vi "motion_control.vi"(2 "position":dbl, 3 "acceleration":dbl, 4 "maxVelocity":dbl, 5 ".NET Refnum in":refnum<k24>) -> (1 ".NET Refnum out":refnum<k24>)   [LabVIEW 2021]
uses:
  C:/Users/User/Documents/Published_files/thorlabs_files/ThorLabs.MotionControl.Benchtop.DCServoCLI.dll
  thorlabs_files/ThorLabs.MotionControl.Benchtop.DCServoCLI.dll
  <vilib>/ptbypt/NI_PtbyPt.lvlib
panel:
  out "end":bool=TRUE
  out "x < y?":bool
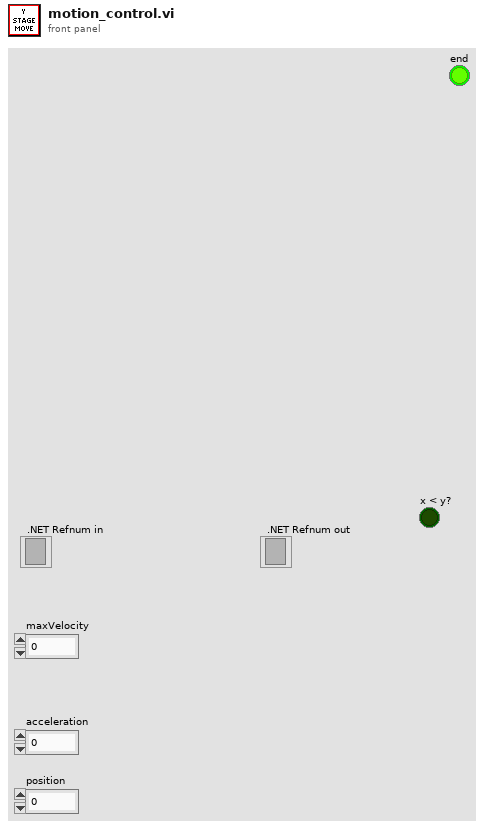
[diagram p1: front panel]
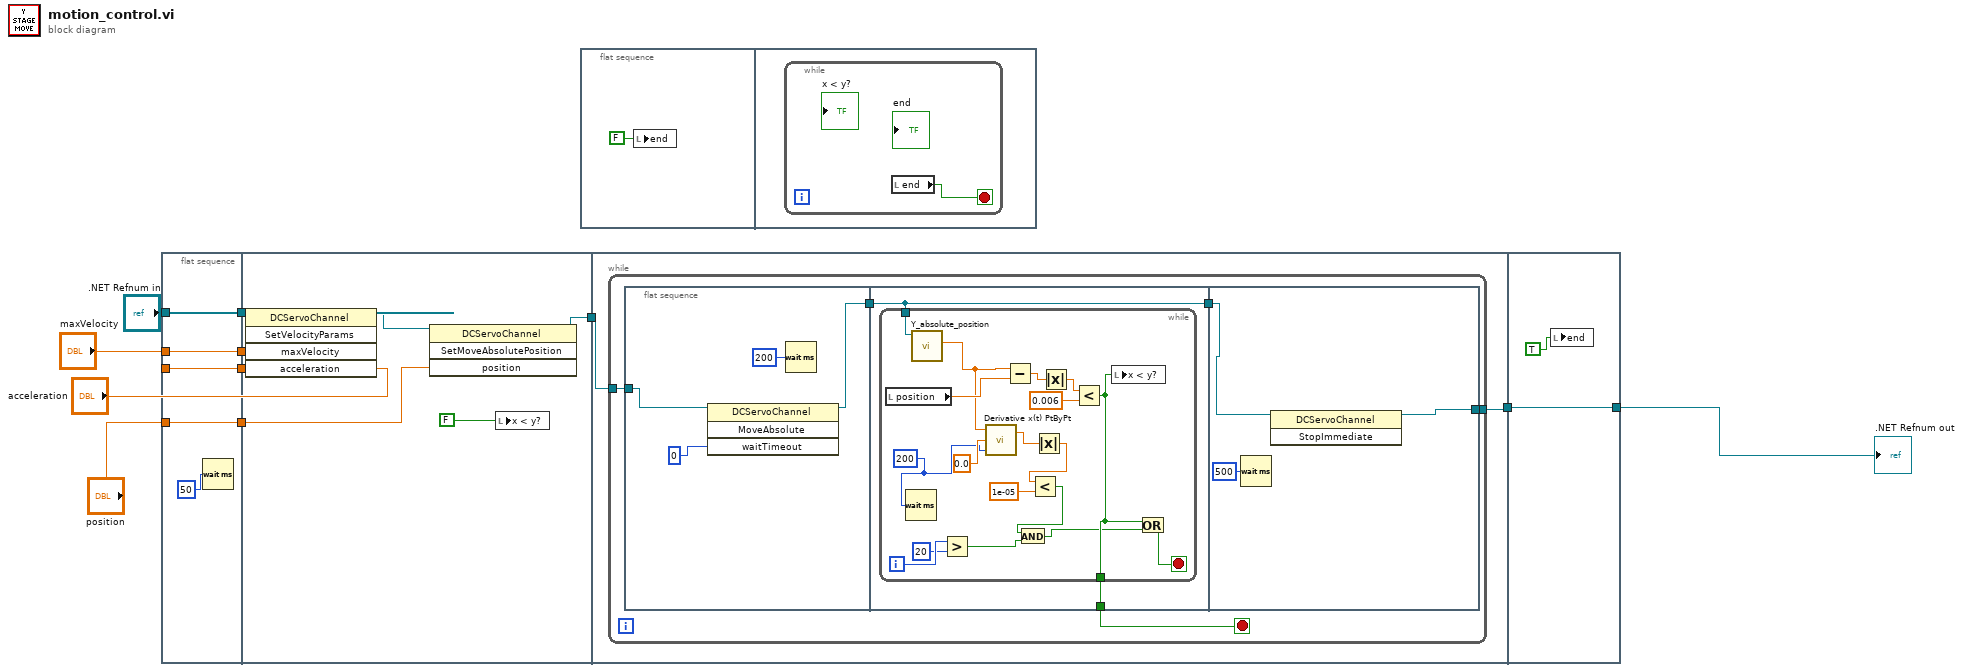
[diagram p0: block diagram]
diagram:
  n1 = flat-sequence {
    tunnel: "maxVelocity" -> [w13]
    tunnel: "acceleration" -> [w14]
    tunnel: "position" -> [w15]
    tunnel: ".NET Refnum in" -> [w16]
    tunnel: [w16] -> w7
    tunnel: [w15] -> w6
    tunnel: [w14] -> w5
    tunnel: [w13] -> w4
    tunnel: w7 -> [w23]
    tunnel: w6 -> [w22]
    tunnel: w5 -> [w21]
    tunnel: w4 -> [w20]
    tunnel: [w17] -> w3
    tunnel: w3 -> [w25]
    tunnel: [w24] -> w1
    tunnel: [w59] -> w2
    tunnel: w1 -> [w59]
    frame #0 {
      n2 = Wait (ms)(milliseconds to wait=u32 50) -> ()  [unwired: 1 out]
    }
    frame #1 {
      n3 = invoke class="DCServoChannel" method="SetVelocityParams"(reference=w23, "maxVelocity"=w20, "acceleration"=w21) -> (reference out=w19:refnum<k24>)  [unwired: 2 in, 4 out]
      n4 = invoke class="DCServoChannel" method="SetMoveAbsolutePosition"(reference=w19, "position"=w22) -> (reference out=w17:refnum<k24>)  [unwired: 2 in, 3 out]
      n5 = local write "x < y?"(FALSE ("x < y? 2")) -> ()
    }
    frame #2 {
      n6 = while {
        tunnel: w25 -> [w30]
        tunnel: [w28] -> w24
        stop <- w29 stop-if-true
        n7 = flat-sequence {
          tunnel: w30 -> [w32]
          tunnel: [w31] -> w26
          tunnel: [w36] -> w29
          tunnel: [w35] -> w27
          tunnel: w26 -> [w35]
          tunnel: [w56] -> w28
          tunnel: w27 -> [w55]
          frame #0 {
            n8 = invoke class="DCServoChannel" method="MoveAbsolute"(reference=w32, "waitTimeout"=0) -> (reference out=w31:refnum<k24>)  [unwired: 2 in, 3 out]
            n9 = Wait (ms)(milliseconds to wait=u32 200) -> ()  [unwired: 1 out]
          }
          frame #1 {
            n10 = while {
              tunnel: [w49] -> w36
              tunnel: w35 -> [w45]
              i -> [w47]
              stop <- w50 stop-if-true
              w41 = u32 200 ("milliseconds to wait")
              n11 = local read "position"() -> (w52:dbl)
              n12 = Wait (ms)(milliseconds to wait=w41) -> ()  [unwired: 1 out]
              n13 = call "Y_absolute_position.vi"(".NET Refnum in"=w45) -> ("Numeric"=w48:dbl)  [unwired: 9 in, 1 out]
              n14 = Greater?(x=w47, y=20) -> (0:w40:bool)
              n15 = call <vilib>:"Derivative x(t) PtByPt.vi"("dt"=w41, "initial condition"=0.0, "x"=w48) -> ("dx/dt"=w38:dbl)  [unwired: 1 in, 1 out]
              n16 = Subtract(x=w48, y=w52) -> (x-y=w53:dbl)
              n17 = Absolute Value(x=w38) -> (abs(x)=w37:dbl)
              n18 = Less?(x=w37, y=1e-05) -> (x < y?=w42:bool)
              n19 = And(x=w42, y=w40) -> (x .and. y?=w39:bool)
              n20 = Absolute Value(x=w53) -> (abs(x)=w54:dbl)
              n21 = Less?(x=w54, y=0.006) -> (x < y?=w49:bool)
              n22 = local write "x < y?"(w49) -> ()
              n23 = Or(x=w49, y=w39) -> (x .or. y?=w50:bool)
            }
          }
          frame #2 {
            n24 = Wait (ms)(milliseconds to wait=u32 500) -> ()  [unwired: 1 out]
            n25 = invoke class="DCServoChannel" method="StopImmediate"(reference=w55) -> (reference out=w56:refnum<k24>)  [unwired: 2 in, 2 out]
          }
        }
      }
    }
    frame #3 {
      n26 = local write "end"(TRUE) -> ()
    }
  }
  n27 = flat-sequence {
    frame #0 {
      n28 = local write "end"(FALSE ("end")) -> ()
    }
    frame #1 {
      n29 = while {
        stop <- w61 stop-if-true
        n30 = local read "end"() -> (w61:bool)
      }
    }
  }
  ".NET Refnum out" <- w2
